vi "LVClass_Pupil Apply Neighbor Extension.vi"(0 "Pupil in":refnum<class "Pupil.lvclass">, 11 "error in (no error)":errorcluster) -> (4 "Pupil out":refnum<class "Pupil.lvclass">, 15 "error out":errorcluster)   [LabVIEW 2020, in "Pupil.lvclass"]
uses:
  Pupil.lvclass
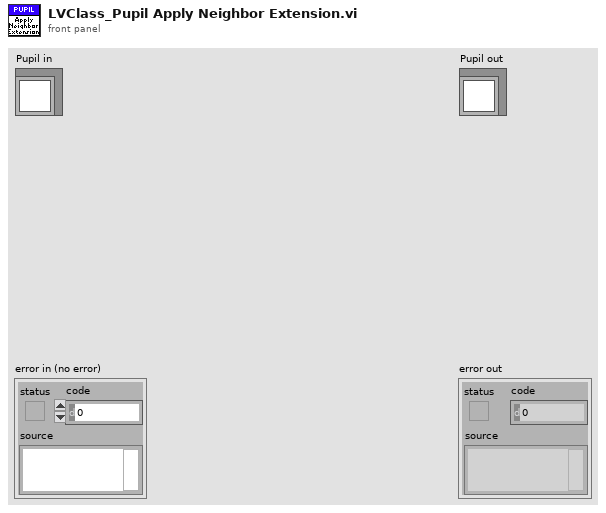
[diagram p1: front panel]
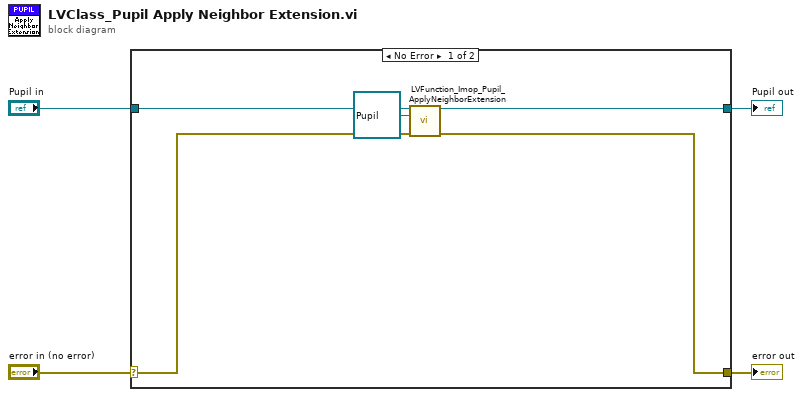
[diagram p0: block diagram]
diagram:
  n1 = case shown="No Error" "error in (no error)" {
    selector: "error in (no error)" -> [w8 w11]
    tunnel: [w7 w11] -> w3
    tunnel: [w6 w10] -> w1
    tunnel: "Pupil in" -> [w9 w10]
    frame No Error {
      n2 = call "LVFunction_Imop_Pupil_ApplyNeighborExtension.vi"("Pupil in"=w9, "Pupil OUT"=refnum<class "Pupil.lvclass"> refnum, "error in (no error)"=w8) -> ("Pupil out"=w6:refnum<class "Pupil.lvclass">, "error out"=w7:errorcluster)  [unwired: 10 in, 1 out]
    }
    frame Error {
    }
  }
  "error out" <- w3
  "Pupil out" <- w1
